vi "Get Lockin Result.vi"(5 "Result in":refnum<class "Acquired Result.lvclass">, 6 "Init work":bool, 7 "Update period":dbl, 8 "error in (no error)":errorcluster, 9 "Last request":bool, 10 "Requester":string, 11 "Lockin Digitizer Driver in":refnum<class "Lockin Digitizer Driver.lvclass">) -> (0 "error out":errorcluster, 1 "Valid result":bool, 2 "Result out":refnum<class "Acquired Result.lvclass">, 3 "Lockin Digitizer Driver out":refnum<class "Lockin Digitizer Driver.lvclass">)   [LabVIEW 2021, in "Lockin Digitizer Driver.lvclass"]
uses:
  Lockin Digitizer Driver.lvclass
  Results/Acquired Result/Acquired Result.lvclass
  Lockin Digitizer Driver.lvclass/Lockin Digitizer Driver.ctl
  <vilib>/express/express signal manip/GetorSetDDTAttributes/Set DDT Attributes/Set DDT Properties.xnode
  <vilib>/express/express shared/transition.llb/Dynamic To Waveform Array.vi
  <vilib>/express/express signal manip/GetorSetDDTAttributes/Set DDT Attributes/SetT0.vi
  <vilib>/express/express shared/transition.llb/Waveform Array To Dynamic.vi
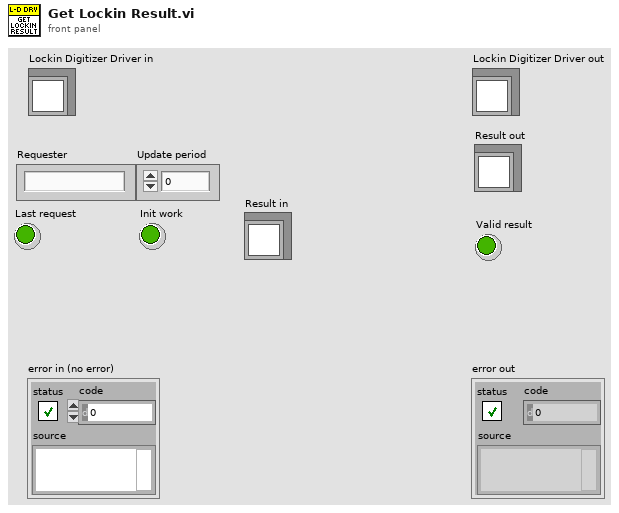
[diagram p1: front panel]
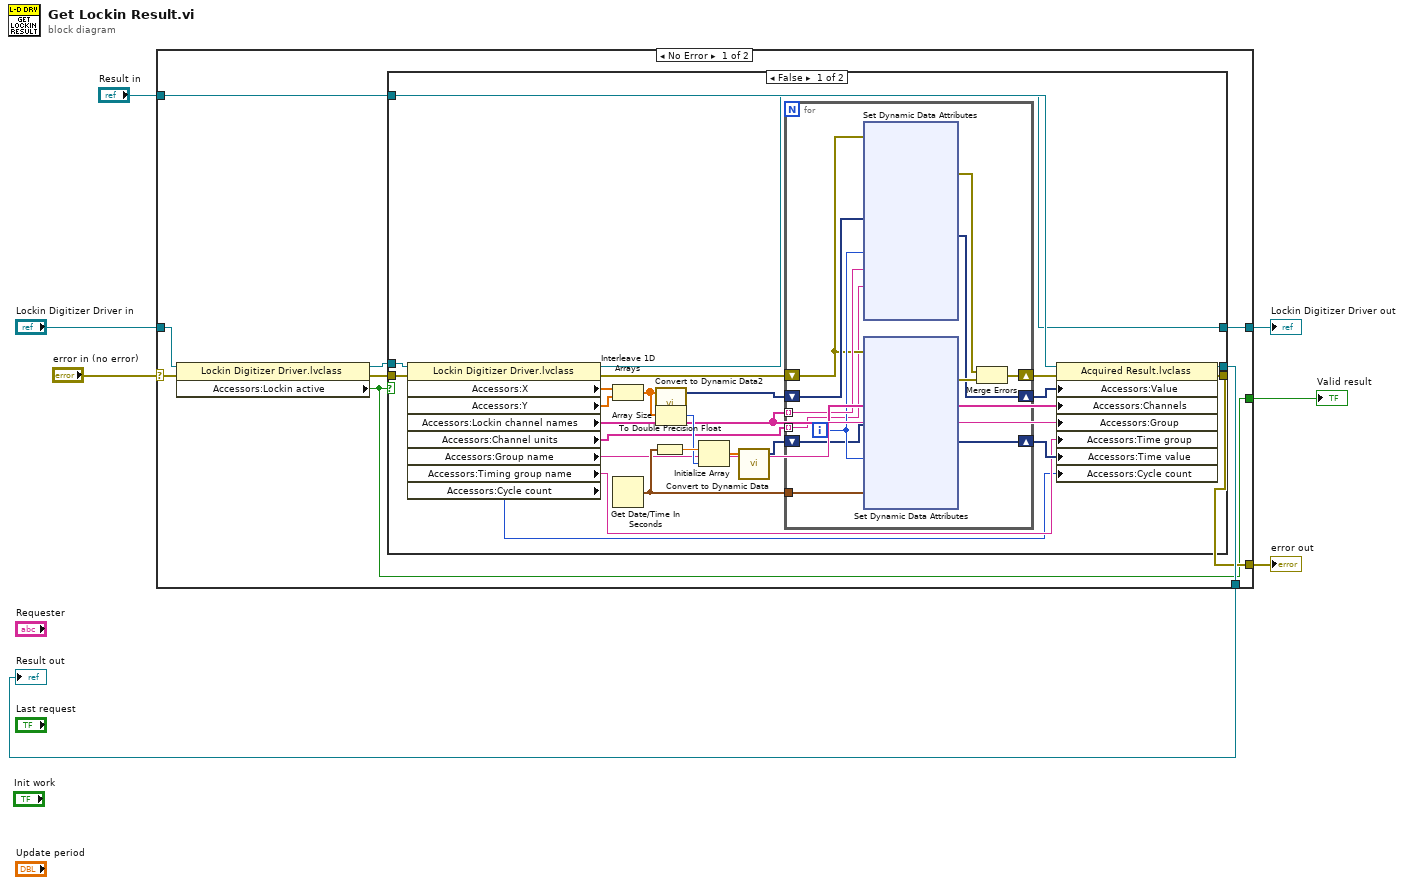
[diagram p0: block diagram]
diagram:
  n1 = case shown="No Error" "error in (no error)" {
    selector: "error in (no error)" -> [w16 w96]
    tunnel: [w10 w96] -> w6
    tunnel: [w9 w95] -> w4
    tunnel: "Lockin Digitizer Driver in" -> [w15 w95]
    tunnel: "Result in" -> [w12 w94]
    tunnel: [w11 w94] -> w2
    tunnel: [w8 _] -> w1
    frame No Error {
      n2 = property class="Lockin Digitizer Driver.lvclass"(reference=w15, error in=w16) -> (reference out=w14:refnum<class "Lockin Digitizer Driver.lvclass">, error out=w13:errorcluster, "Accessors:Lockin active"=w8:bool)
      n3 = case shown="False" w8 {
        tunnel: w14 -> [w40 w92]
        tunnel: w13 -> [w39 w91]
        tunnel: w12 -> [w27 w93]
        tunnel: [w19 w93] -> w11
        tunnel: [w18 w91] -> w10
        tunnel: [w17 w92] -> w9
        frame False {
          n4 = property class="Lockin Digitizer Driver.lvclass"(reference=w40, error in=w39) -> (reference out=w17:refnum<class "Lockin Digitizer Driver.lvclass">, error out=w29:errorcluster, "Accessors:X"=w33:dbl[], "Accessors:Y"=w32:dbl[], "Accessors:Lockin channel names"=w21:string[], "Accessors:Channel units"=w28:string[], "Accessors:Group name"=w22:string, "Accessors:Timing group name"=w23:string, "Accessors:Cycle count"=w20:i32)
          n5 = Interleave 1D Arrays(w33, w32) -> (w31:dbl[])
          n6 = Get Date/Time In Seconds() -> (seconds since 1Jan1904=w35:timestamp)
          n7 = To Double Precision Float(number=w35) -> (double precision float=w38:dbl)
          n8 = call "Convert to Dynamic Data2"("Array"=w31) -> ("Dynamic Data Type"=w34:dynamicdata)  [unwired: 3 in]
          n9 = Array Size(array=w31) -> (size(s)=w36:i32)
          n10 = Initialize Array(w38, w36) -> (w37:dbl[])
          n11 = call "Convert to Dynamic Data"("Array"=w37) -> ("Dynamic Data Type"=w30:dynamicdata)  [unwired: 3 in]
          n12 = for {
            tunnel: w21 -> [w52] mode=indexing
            shift-right: [w41] -> w25
            shift-left: w34 -> [w49]
            tunnel: w35 -> [w51]
            shift-right: [w42] -> w24
            shift-left: w30 -> [w48]
            shift-right: [w46] -> w26
            shift-left: w29 -> [w44]
            tunnel: w28 -> [w43] mode=indexing
            i -> [w50]
            n13 = xnode "Set Dynamic Data Attributes"("Signals In"=w49, "Signal Index"=w50, "Signal Name"=w52, "Unit"=w43, "error in"=w44) -> ("Signals Out"=w41:dynamicdata, "error out"=w47:errorcluster)  [unwired: 1 in]
            n14 = xnode "Set Dynamic Data Attributes"("Signals In"=w48, "Signal Index"=w50, "Timestamp"=w51, "error in"=w44) -> ("Signals Out"=w42:dynamicdata, "error out"=w45:errorcluster)  [unwired: 1 in]
            n15 = Merge Errors(w47, w45) -> (w46:errorcluster)
          }
          n16 = property class="Acquired Result.lvclass"(reference=w27, error in=w26, "Accessors:Value"=w25, "Accessors:Channels"=w21, "Accessors:Group"=w22, "Accessors:Time group"=w23, "Accessors:Time value"=w24, "Accessors:Cycle count"=w20) -> (reference out=w19:refnum<class "Acquired Result.lvclass">, error out=w18:errorcluster)
        }
        frame True {
        }
      }
    }
    frame Error {
    }
  }
  "error out" <- w6
  "Lockin Digitizer Driver out" <- w4
  "Result out" <- w2
  "Valid result" <- w1
